vi "Get Oldest Time to Plot.vi"(1 "History Length":dbl=1800.0 format="%<%M:%S>t", 2 "Clear Plot":bool) -> (0 "Oldest Time to Plot":dbl)   [LabVIEW 2012]
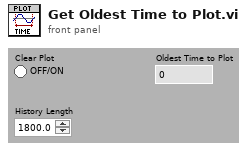
[diagram p1: front panel]
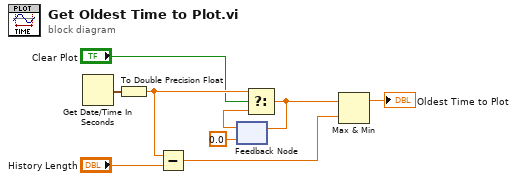
[diagram p0: block diagram]
diagram:
  n1 = Get Date/Time In Seconds() -> (seconds since 1Jan1904=w2:timestamp)
  n2 = To Double Precision Float(number=w2) -> (double precision float=w5:dbl)
  n3 = Subtract(x=w5, y="History Length") -> (x-y=w8:dbl)
  n4 = feedback #1(0.0) -> (w6:dbl)
  n5 = Select(t=w5, s="Clear Plot", f=w6) -> (s? t:f=w7:dbl)
  n6 = feedback-in #1(w7) -> ()
  n7 = Max & Min(x=w7, y=w8) -> (max(x,y)=→"Oldest Time to Plot":dbl)  [unwired: 1 out]
